vi "Write IP Address.vi"(10 "IP Address":string, 11 "UDP Listener in":refnum<class "UDP Listener.lvclass">) -> (3 "UDP Listener out":refnum<class "UDP Listener.lvclass">)   [LabVIEW 2016, in "Assert Service.lvlib" / "UDP Listener.lvclass"]
uses:
  UDP Listener.lvclass
  UDP Listener.lvclass/UDP Listener.ctl
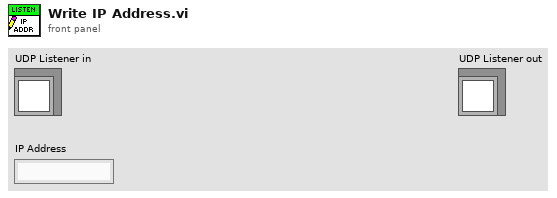
[diagram p1: front panel]
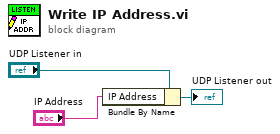
[diagram p0: block diagram]
diagram:
  n1 = Bundle By Name(cluster="UDP Listener in", "IP Address"="IP Address") -> (→"UDP Listener out":refnum<class "UDP Listener.lvclass">)
